vi "Finish.vi"   [LabVIEW 2020]
doc: "This VI is called just before exiting. It is expected to close I/O refnum, save collected data, etc."
uses:
  <vilib>/Rock Robotics/WPI/Utilities/WPI_GetSetVariantRefNum.vi
types:
  T1 = typedef "WPI_MotorControlDeviceRef.ctl" = cluster{"DeviceStatus":errorcluster, "Type":T2, "PWM":cluster{"PWM Channel":T3, "DeadBand":T4}, "CAN":cluster{"Device Number":u8, "SetOutput VI Ref":variant, "GetOutput VI Ref":variant, "Enable VI Ref":variant, "Disable VI Ref":variant, "Data":variant}, "Invert":bool, "DIO PWM":cluster{"PWM \"Enable\" Channel":T3, "DIOChannel":T5, "PWM Rate":dbl}}
  T2 = typedef "WPI_MotorControlType.ctl" = enum16{"PWM", "CAN", "DIO PWM"}
  T3 = typedef "FPGA_DIOPWMChannel.ctl" = enum8{"PWM 0", "PWM 1", "PWM 2", "PWM 3", "PWM 4", "PWM 5", "PWM 6", "PWM 7", "PWM 8", "PWM 9", "PWM MXP 0", "PWM MXP 1", "PWM MXP 2", "PWM MXP 3", "PWM MXP 4", "PWM MXP 5", "PWM MXP 6", "PWM MXP 7", "PWM MXP 8", "PWM MXP 9", "Invalid"}
  T4 = typedef "WPI_PWMDeadband.ctl" = cluster{"Name":string, "maxPositivePwm":i32, "minPositivePwm":i32, "centerPwm":i32, "maxNegativePwm":i32, "minNegativePwm":i32, "angularRange":u16}
  T5 = typedef "FPGA_DIOChannel.ctl" = enum8{"DIO 0", "DIO 1", "DIO 2", "DIO 3", "DIO 4", "DIO 5", "DIO 6", "DIO 7", "DIO 8", "DIO 9", "DIO MXP 0", "DIO MXP 1", "DIO MXP 2", "DIO MXP 3", "DIO MXP 4", "DIO MXP 5", "DIO MXP 6", "DIO MXP 7", "DIO MXP 8", "DIO MXP 9", "DIO MXP 10", "DIO MXP 11", "DIO MXP 12", "DIO MXP 13", "DIO MXP 14", "DIO MXP 15", "SPI Port CS1", "SPI Port CS2", "SPI Port CS3", "SPI Port MISO", "SPI Port MOSI", "Invalid"}
  T6 = typedef "WPI_SwitchDevRef.ctl" = cluster{"DevStatus":errorcluster, "DIO Channel":T5, "CntIndex":T7, "Normally Closed":bool}
  T7 = typedef "FPGA_CounterCtrSystemIndex.ctl" = enum8{"Ctr 0", "Ctr 1", "Ctr 2", "Ctr 3", "Ctr 4", "Ctr 5", "Ctr 6", "Ctr 7", "Invalid"}
  T8 = typedef "WPI_GyroDevRef.ctl" = cluster{"DevStatus":errorcluster, "Analog Channel":T9, "Gain (VoltsPerDegree/Second)":dbl, "Gyro Type":enum16{"Analog", "XRS450"}, "Handle":i32, "SPI Bus":T10, "Device Found":bool, "Sample Rate":dbl, "Calibrate On Open":bool, "Offset":dbl}
  T9 = typedef "FPGA_AIChannel.ctl" = enum8{"AI 0", "AI 1", "AI 2", "AI 3", "AI MXP 0", "AI MXP 1", "AI MXP 2", "AI MXP 3", "Invalid"}
  T10 = typedef "spi_bus.ctl" = enum16{"SPI On-Board, CS0", "SPI On-Board, CS1", "SPI On-Board, CS2", "SPI On-Board, CS3", "SPI MXP", "Invalid"}
  T11 = typedef "WPI_JoystickDevRef.ctl" = cluster{"Device":T12}
  T12 = typedef "WPI_JoystickDeviceEnum.ctl" = enum16{"USB 0", "USB 1", "USB 2", "USB 3", "USB 4", "USB 5"}
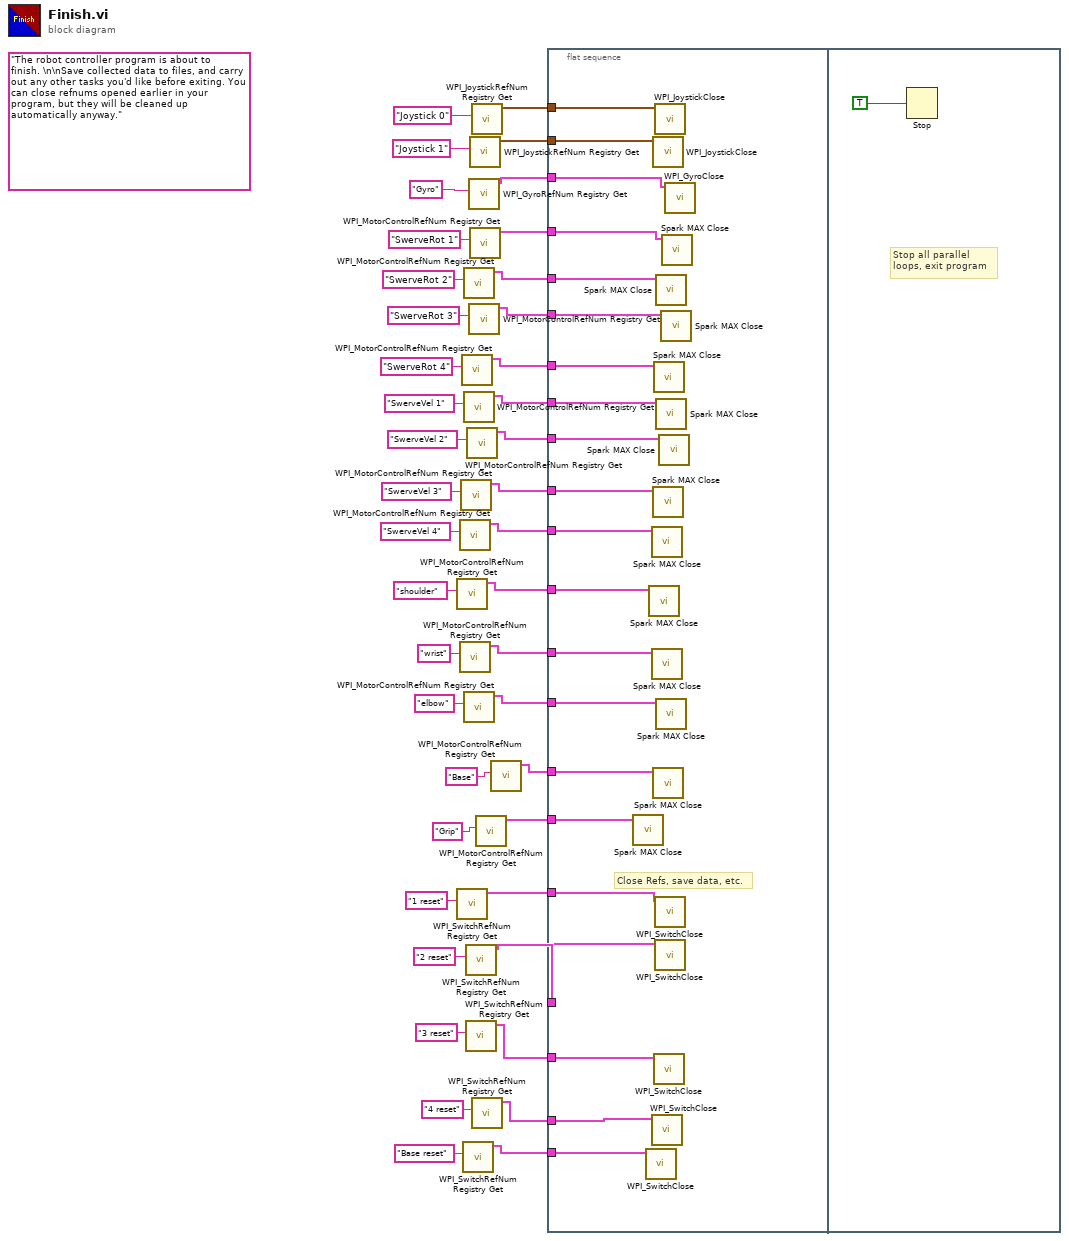
[diagram p0: block diagram]
diagram:
  (unwired) "The robot controller program is about to finish. \n\nSave collected data to files, and carry out any other tasks you'd like before exiting. You can close refnums opened earlier in your program, but they will be cleaned up automatically anyway."
  n1 = call <vilib>:"WPI_MotorControlRefNum Registry Get.vi"("refnum name"="shoulder") -> ("MotorControlDevRef"=w22:T1)  [unwired: 9 in, 1 out]
  n2 = call <vilib>:"WPI_SwitchRefNum Registry Get.vi"("refnum name"="1 reset") -> ("SwitchDevRef"=w13:T6)  [unwired: 9 in, 1 out]
  n3 = call <vilib>:"WPI_MotorControlRefNum Registry Get.vi"("refnum name"="SwerveVel 4") -> ("MotorControlDevRef"=w23:T1)  [unwired: 9 in, 1 out]
  n4 = call <vilib>:"WPI_MotorControlRefNum Registry Get.vi"("refnum name"="wrist") -> ("MotorControlDevRef"=w19:T1)  [unwired: 9 in, 1 out]
  n5 = call <vilib>:"WPI_MotorControlRefNum Registry Get.vi"("refnum name"="SwerveVel 3") -> ("MotorControlDevRef"=w24:T1)  [unwired: 9 in, 1 out]
  n6 = call <vilib>:"WPI_MotorControlRefNum Registry Get.vi"("refnum name"="SwerveRot 4") -> ("MotorControlDevRef"=w27:T1)  [unwired: 9 in, 1 out]
  n7 = call <vilib>:"WPI_SwitchRefNum Registry Get.vi"("refnum name"="Base reset") -> ("SwitchDevRef"=w1:T6)  [unwired: 9 in, 1 out]
  n8 = call <vilib>:"WPI_MotorControlRefNum Registry Get.vi"("refnum name"="SwerveRot 2") -> ("MotorControlDevRef"=w29:T1)  [unwired: 9 in, 1 out]
  n9 = call <vilib>:"WPI_MotorControlRefNum Registry Get.vi"("refnum name"="SwerveVel 1") -> ("MotorControlDevRef"=w26:T1)  [unwired: 9 in, 1 out]
  n10 = call <vilib>:"WPI_MotorControlRefNum Registry Get.vi"("refnum name"="elbow") -> ("MotorControlDevRef"=w18:T1)  [unwired: 9 in, 1 out]
  n11 = call <vilib>:"WPI_SwitchRefNum Registry Get.vi"("refnum name"="2 reset") -> ("SwitchDevRef"=w9:T6)  [unwired: 9 in, 1 out]
  n12 = call <vilib>:"WPI_SwitchRefNum Registry Get.vi"("refnum name"="3 reset") -> ("SwitchDevRef"=w8:T6)  [unwired: 9 in, 1 out]
  n13 = call <vilib>:"WPI_MotorControlRefNum Registry Get.vi"("refnum name"="SwerveVel 2") -> ("MotorControlDevRef"=w25:T1)  [unwired: 9 in, 1 out]
  n14 = call <vilib>:"WPI_GyroRefNum Registry Get.vi"("refnum name"="Gyro") -> ("GyroDevRef"=w31:T8)  [unwired: 9 in, 1 out]
  n15 = call <vilib>:"WPI_MotorControlRefNum Registry Get.vi"("refnum name"="SwerveRot 3") -> ("MotorControlDevRef"=w28:T1)  [unwired: 9 in, 1 out]
  n16 = call <vilib>:"WPI_JoystickRefNum Registry Get.vi"("refnum name"="Joystick 1") -> ("JoystickDevRef"=w16:T11)  [unwired: 1 in, 9 out]
  n17 = call <vilib>:"WPI_MotorControlRefNum Registry Get.vi"("refnum name"="SwerveRot 1") -> ("MotorControlDevRef"=w30:T1)  [unwired: 9 in, 1 out]
  n18 = call <vilib>:"WPI_JoystickRefNum Registry Get.vi"("refnum name"="Joystick 0") -> ("JoystickDevRef"=w41:T11)  [unwired: 1 in, 9 out]
  n19 = call <vilib>:"WPI_SwitchRefNum Registry Get.vi"("refnum name"="4 reset") -> ("SwitchDevRef"=w7:T6)  [unwired: 9 in, 1 out]
  n20 = call <vilib>:"WPI_MotorControlRefNum Registry Get.vi"("refnum name"="Grip") -> ("MotorControlDevRef"=w3:T1)  [unwired: 9 in, 1 out]
  n21 = call <vilib>:"WPI_MotorControlRefNum Registry Get.vi"("refnum name"="Base") -> ("MotorControlDevRef"=w5:T1)  [unwired: 9 in, 1 out]
  n22 = flat-sequence {
    tunnel: w41 -> [w63]
    tunnel: w31 -> [w62]
    tunnel: w30 -> [w61]
    tunnel: w29 -> [w60]
    tunnel: w28 -> [w59]
    tunnel: w27 -> [w58]
    tunnel: w26 -> [w57]
    tunnel: w25 -> [w56]
    tunnel: w24 -> [w55]
    tunnel: w23 -> [w54]
    tunnel: w22 -> [w53]
    tunnel: w19 -> [w52]
    tunnel: w18 -> [w51]
    tunnel: w16 -> [w50]
    tunnel: w13 -> [w49]
    tunnel: w9 -> [w48]
    tunnel: w8 -> [w47]
    tunnel: w7 -> [w46]
    tunnel: w5 -> [w45]
    tunnel: w3 -> [w44]
    tunnel: w1 -> [w43]
    frame #0 {
      # "Close Refs, save data, etc."
      n23 = call <vilib>:"Spark MAX Close.vi"("MotorControlDeviceRef"=w44) -> ()  [unwired: 10 in, 1 out]
      n24 = call <vilib>:"WPI_SwitchClose.vi"("SwitchDevRef"=w43) -> ()  [unwired: 10 in, 1 out]
      n25 = call <vilib>:"Spark MAX Close.vi"("MotorControlDeviceRef"=w53) -> ()  [unwired: 10 in, 1 out]
      n26 = call <vilib>:"Spark MAX Close.vi"("MotorControlDeviceRef"=w54) -> ()  [unwired: 10 in, 1 out]
      n27 = call <vilib>:"Spark MAX Close.vi"("MotorControlDeviceRef"=w52) -> ()  [unwired: 10 in, 1 out]
      n28 = call <vilib>:"WPI_SwitchClose.vi"("SwitchDevRef"=w46) -> ()  [unwired: 10 in, 1 out]
      n29 = call <vilib>:"WPI_JoystickClose.vi"("JoystickDevRef"=w50) -> ()  [unwired: 11 out]
      n30 = call <vilib>:"Spark MAX Close.vi"("MotorControlDeviceRef"=w55) -> ()  [unwired: 10 in, 1 out]
      n31 = call <vilib>:"Spark MAX Close.vi"("MotorControlDeviceRef"=w45) -> ()  [unwired: 10 in, 1 out]
      n32 = call <vilib>:"Spark MAX Close.vi"("MotorControlDeviceRef"=w58) -> ()  [unwired: 10 in, 1 out]
      n33 = call <vilib>:"WPI_SwitchClose.vi"("SwitchDevRef"=w47) -> ()  [unwired: 10 in, 1 out]
      n34 = call <vilib>:"WPI_JoystickClose.vi"("JoystickDevRef"=w63) -> ()  [unwired: 11 out]
      n35 = call <vilib>:"WPI_SwitchClose.vi"("SwitchDevRef"=w49) -> ()  [unwired: 10 in, 1 out]
      n36 = call <vilib>:"WPI_SwitchClose.vi"("SwitchDevRef"=w48) -> ()  [unwired: 10 in, 1 out]
      n37 = call <vilib>:"Spark MAX Close.vi"("MotorControlDeviceRef"=w60) -> ()  [unwired: 10 in, 1 out]
      n38 = call <vilib>:"Spark MAX Close.vi"("MotorControlDeviceRef"=w57) -> ()  [unwired: 10 in, 1 out]
      n39 = call <vilib>:"Spark MAX Close.vi"("MotorControlDeviceRef"=w51) -> ()  [unwired: 10 in, 1 out]
      n40 = call <vilib>:"Spark MAX Close.vi"("MotorControlDeviceRef"=w56) -> ()  [unwired: 10 in, 1 out]
      n41 = call <vilib>:"Spark MAX Close.vi"("MotorControlDeviceRef"=w59) -> ()  [unwired: 10 in, 1 out]
      n42 = call <vilib>:"Spark MAX Close.vi"("MotorControlDeviceRef"=w61) -> ()  [unwired: 10 in, 1 out]
      n43 = call <vilib>:"WPI_GyroClose.vi"("GyroDevRef"=w62) -> ()  [unwired: 10 in, 1 out]
    }
    frame #1 {
      # "Stop all parallel\nloops, exit program"
      n44 = Stop(stop? (T)=TRUE ("Quit")) -> ()
    }
  }
